vi "GV photoncounter input selector.vi"() -> ()   [LabVIEW 2017]
panel:
  out "PhotoncounterInputSelector":u8
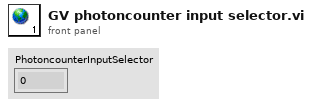
[diagram p1: front panel]
diagram:
